vi "Request Data.vi"(10 "Elements remain?":bool, 11 "Address counter":u32) -> (3 "Address counter output":u32)   [LabVIEW 2015]
uses:
  <vilib>/rvi/Memory/Memory_Emulation/niFpgaMemoryEmulationDramWriteAndRequestData.vi
  <vilib>/rvi/Memory/Memory_Emulation/niFpgaMemoryFastEmulationDramWriteAndRequestData.vi
  <vilib>/rvi/DataTransferAndStorage/Container/Common/niFpgaContainerGetUniqueNameForEmu.vi
  <vilib>/rvi/Memory/Memory_Emulation/niFpgaMemoryEmulationCacheClearOnFirstRun.vi
  <vilib>/rvi/Memory/Memory_Emulation/nirvimemoryEmulationManagerCache_MakeExclusive.vi
  <vilib>/rvi/Memory/Memory_Emulation/nirvimemoryEmulationManagerCache_GetValue.vi
  <vilib>/rvi/Memory/Memory_Emulation/nirvimemoryEmulationManagerCache_InsertValue.vi
  <vilib>/Utility/error.llb/Clear Errors.vi
  <vilib>/rvi/Memory/Memory_Emulation/nirvimemoryEmulationManagerCache_ReleaseExclusive.vi
  <vilib>/rvi/Memory/Memory_Emulation/niFpgaMemoryEmulationDramWriteAndRequestDataApplyByteEnables.vi
  <vilib>/rvi/Memory/Memory_Emulation/nirvimemoryEmulationManagerCache_SetValue.vi
  <vilib>/rvi/DataTransferAndStorage/Container/XNode/niFpgaContainer.xnode
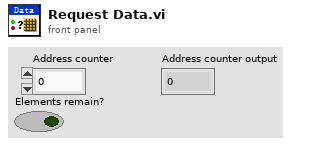
[diagram p1: front panel]
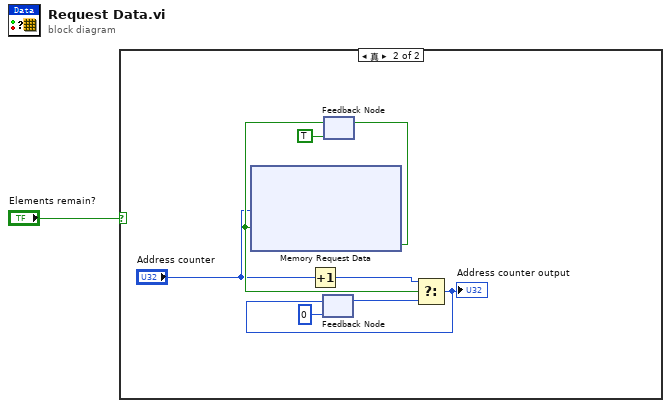
[diagram p0: block diagram]
diagram:
  n1 = case shown="真" "Elements remain?" {
    frame False {
    }
    frame True {
      n2 = Increment(x="Address counter") -> (x+1=w7:u32)
      n3 = feedback #1(u32 0) -> (w5:u32)
      n4 = feedback #2(TRUE ("Ready for Input")) -> (w4:bool)
      n5 = xnode ("Memory Request Data")("地址"="Address counter", "输入有效"=w4) -> ("输入就绪"=w2:bool)  [unwired: 1 in, 1 out]
      n6 = feedback-in #2(w2) -> ()
      n7 = Select(t=w7, s=w4, f=w5) -> (s? t:f=w6:u32)
      "Address counter output" <- w6
      n8 = feedback-in #1(w6) -> ()
    }
  }
